vi "randompassword.vi"() -> (0 "Password":string)   [LabVIEW 2024]
uses:
  <vilib>/numeric/Random Number (Range) U64.vi
  <vilib>/numeric/sub_Random U32.vi
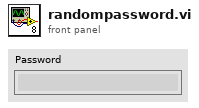
[diagram p1: front panel]
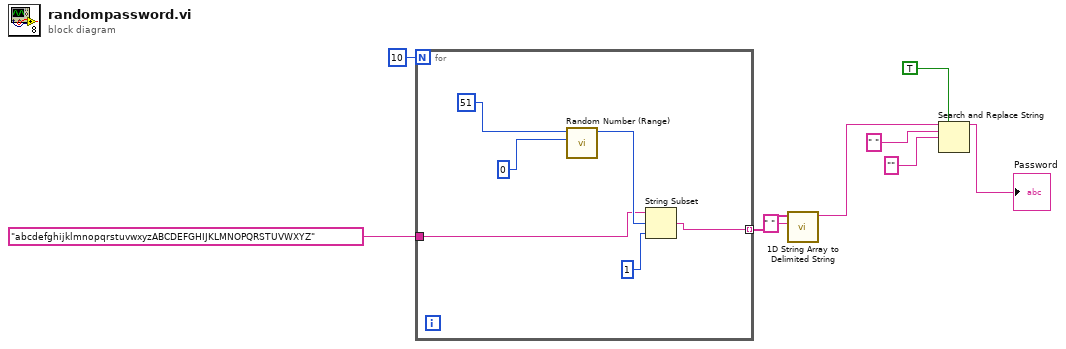
[diagram p0: block diagram]
diagram:
  n1 = for {
    N: 10 -> [_]
    tunnel: "abcdefghijklmnopqrstuvwxyzABCDEFGHIJKLMNOPQRSTUVWXYZ" -> [w12]
    tunnel: [w11] -> w7 mode=indexing
    n2 = call-poly <vilib>:"Random Number (Range).vi"("lower bound (0)"=u64 0, "upper bound (100)"=u64 51) -> ("number"=w13:u64)  [unwired: 9 in]
    n3 = String Subset(string=w12, offset (0)=w13, length (rest)=1 ("length (rest)")) -> (substring=w11:string)
  }
  n4 = call <vilib>:"1D String Array to Delimited String.vi"("delimiter"=" ", "string array"=w7) -> ("delimited string"=w4:string)  [unwired: 9 in]
  n5 = Search and Replace String(replace all?=TRUE, input string=w4, search string=" ", replace string="" ("replace string (\"\")")) -> (result string=→"Password":string)  [unwired: 4 in, 3 out]
